vi "LSX Get Snapshot Filter.vi"(8 "error in (no error)":errorcluster, 10 "plTime":i32, 11 "lLSID":i32) -> (0 "error out":errorcluster, 2 "plTime out":i32, 3 "function return":i32)   [LabVIEW 2018, in "Tango.lvlib"]
doc: "TANGOAPI int TANGOCALL LSX_GetSnapshotFilter (int lLSID, int *plTime);"
uses:
  Tango.lvlib
  SubVIs/Tango_DLL.dll
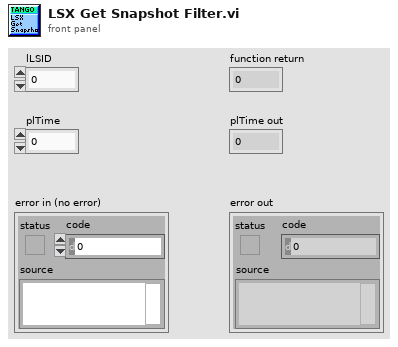
[diagram p1: front panel]
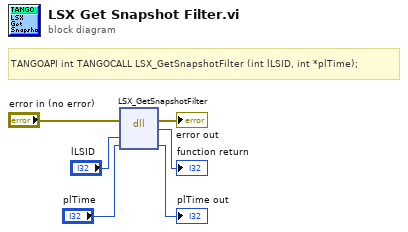
[diagram p0: block diagram]
diagram:
  # "TANGOAPI int TANGOCALL LSX_GetSnapshotFilter (int lLSID, int *plTime);"
  n1 = dll-call lib="C:/Users/Familie/Documents/LabviewIX81/lib/TANGO Stage/SubVIs/Tango_DLL.*" fn="LSX_GetSnapshotFilter"(error in="error in (no error)", "lLSID"="lLSID", "plTime"="plTime") -> (error out=→"error out":errorcluster, →"function return":i32, "plTime"=→"plTime out":i32)  [unwired: 3 in, 1 out]
